vi "ABFImport_Open.vi"(8 "error in (no error)":errorcluster, 11 "abf file path":path) -> (0 "error out":errorcluster, 3 "reference number":i32)   [LabVIEW 2017]
uses:
  LV_ABFIO.dll
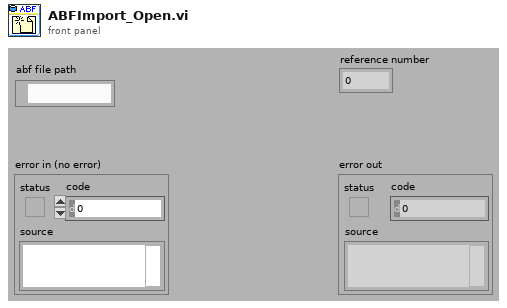
[diagram p1: front panel]
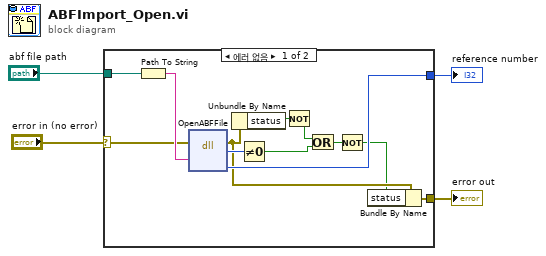
[diagram p0: block diagram]
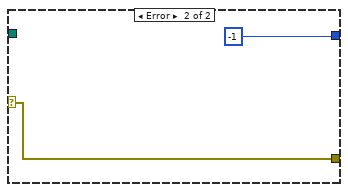
[diagram p2: hidden frame]
diagram:
  n1 = case shown="에러 없음" "error in (no error)" {
    selector: "error in (no error)" -> [w14 w17]
    tunnel: [w13 -1] -> w3
    tunnel: "abf file path" -> [w16 _]
    tunnel: [w5 w17] -> w1
    frame No Error {
      n2 = Path To String(path=w16) -> (string=w15:string)
      n3 = dll-call lib="C:/Users/KimYG/Application/Solution Package/APIs/LV_ABFIO.dll" fn="OpenABFFile"(error in=w14, "arg1"=w15) -> (error out=w8:errorcluster, "return type"=w12:i32, "arg3"=w13:i32)  [unwired: 4 in, 1 out]
      n4 = Unbundle By Name(w8) -> ("status"=w11:bool)
      n5 = Not Equal To 0?(x=w12) -> (x != 0?=w9:bool)
      n6 = Not(x=w11) -> (.not. x?=w10:bool)
      n7 = Or(x=w10, y=w9) -> (x .or. y?=w7:bool)
      n8 = Not(x=w7) -> (.not. x?=w6:bool)
      n9 = Bundle By Name(cluster=w8, "status"=w6) -> (w5:errorcluster)
    }
    frame Error {
    }
  }
  "error out" <- w1
  "reference number" <- w3
